vi "RealSense_HelloWorld_Left_Right_IR.vi"() -> ()   [LabVIEW 2017]
doc: "This demo shows how to connect a RealSense D4xx Stereo Depth Camera, and stream the LEFT and the RIGHT raw unrectified images."
uses:
  libRealSense3.lvlib
panel:
  in  "Zoom Factor":sgl
  in  "AutoZoom":bool
  out "Output stream format":T1
  in  "laser on/off":bool
  out "Left IR":picture
  out "Right IR":picture
  out "iteration":i32
  in  "stop":bool=TRUE
  out "release frame error":string="No Error"
  out "Capture1 Error":string="No Error"
  out "Config error":string="No Error\rNo Error"
  out "init results":T2={"camera name"="Intel RealSense 415", "camera S/N"="725112060291", "F/W"="05.08.09.00", "Sensor name"="Stereo Module", "api_version"=20710, "rscontext"=659718592, "device_list"=396628960, "device count"=2, "Dev out"=662505184, "sensor_list"=395031584, "sensor count"=2, "Sensor out"=662178704}
  out "init error":string="No Error\rNo Error\rNo Error\rNo Error\rNo Error\rNo Error\rNo Error\rNo Error\rNo Error\rNo Error\rNo Error"
  out "Close Error":string="No Error\rNo Error\rNo Error\rNo Error"
  out "Start Error":string="No Error\rNo Error\rNo Error"
  out "Capture2 error":string="No Error"
  in  "Select Resolution":u16(ring)=3 items=["256 x 144 @90fps", "424 x 240 @6fps", "424 x 240 @15fps", "424 x 240 @30fps", "424 x 240 @60fps", "424 x 240 @90fps", "480 x 270 @6fps", "480 x 270 @15fps", "480 x 270 @30fps", "480 x 270 @60fps", "480 x 270 @90fps", "640 x 360 @6fps", "640 x 360 @15fps", "640 x 360 @30fps", "640 x 360 @60fps", "640 x 360 @90fps", "640 x 480 @6fps", "640 x 480 @15fps", "640 x 480 @30fps", "640 x 480 @60fps", "640 x 480 @90fps", "848 x 100 @100fps", "848 x 480 @6fps", "848 x 480 @15fps", "848 x 480 @30fps", "848 x 480 @60fps", "848 x 480 @90fps", "1280 x 720 @6fps", "1280 x 720 @15fps", "1280 x 720 @30fps", "1280 x 800 @15fps", "1280 x 800 @30fps"]
  # "RealSense Hello World: Left-Right Rectified"
  # "This demo shows how to connect a RealSense D4xx Stereo Depth Camera, and stream the LEFT and the RIGHT images."
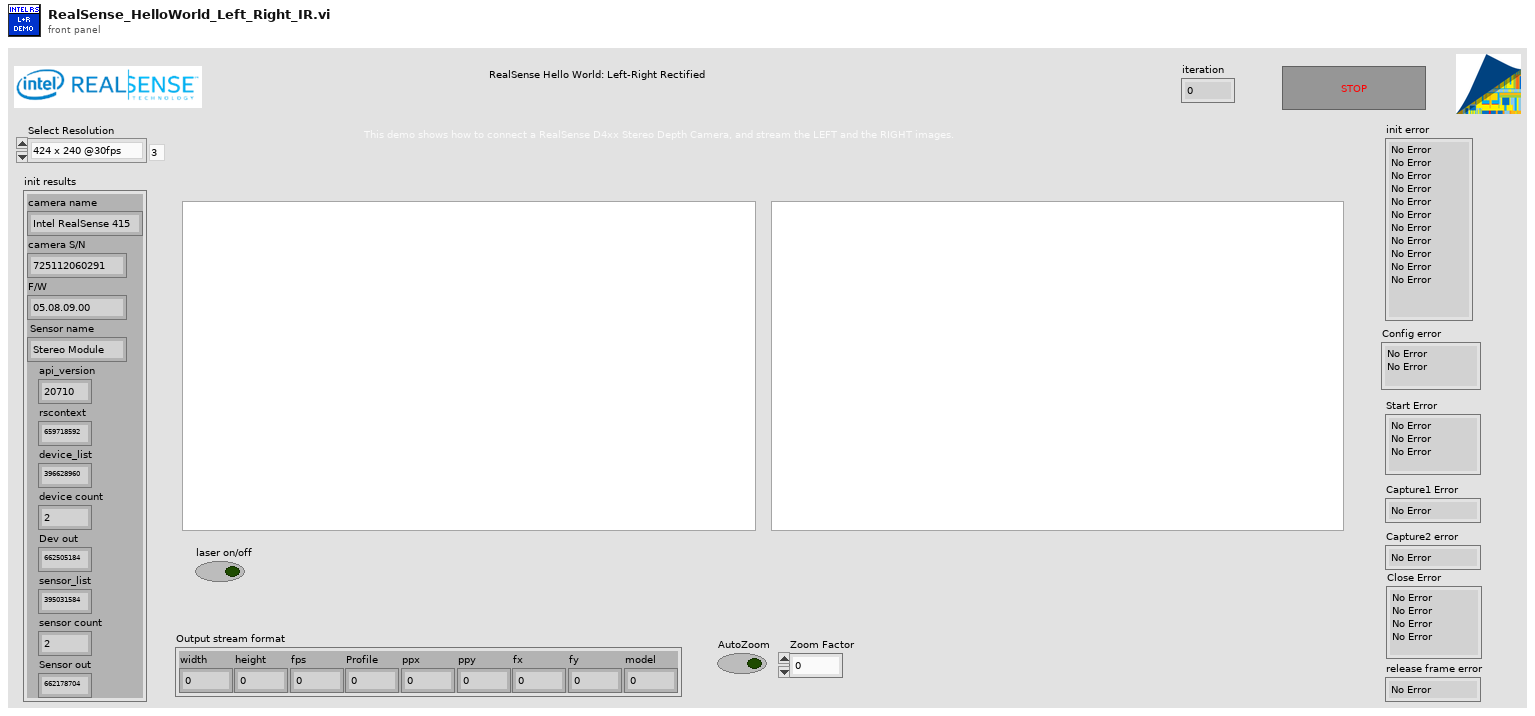
[diagram p1: front panel]
types:
  T1 = cluster{"width":i32, "height":i32, "fps":i32, "Profile":u64, "ppx":sgl, "ppy":sgl, "fx":sgl, "fy":sgl, "model":u32}
  T2 = cluster{"camera name":string, "camera S/N":string, "F/W":string, "Sensor name":string, "api_version":i32, "rscontext":u64, "device_list":u64, "device count":i32, "Dev out":u64, "sensor_list":u64, "sensor count":i32, "Sensor out":u64}
  T3 = enum16{"Depth", "Color (ext.)", "Color (left) ", "IR Left", "IR Right", "IR Left (Y16)", "IR Right (Y16)"}
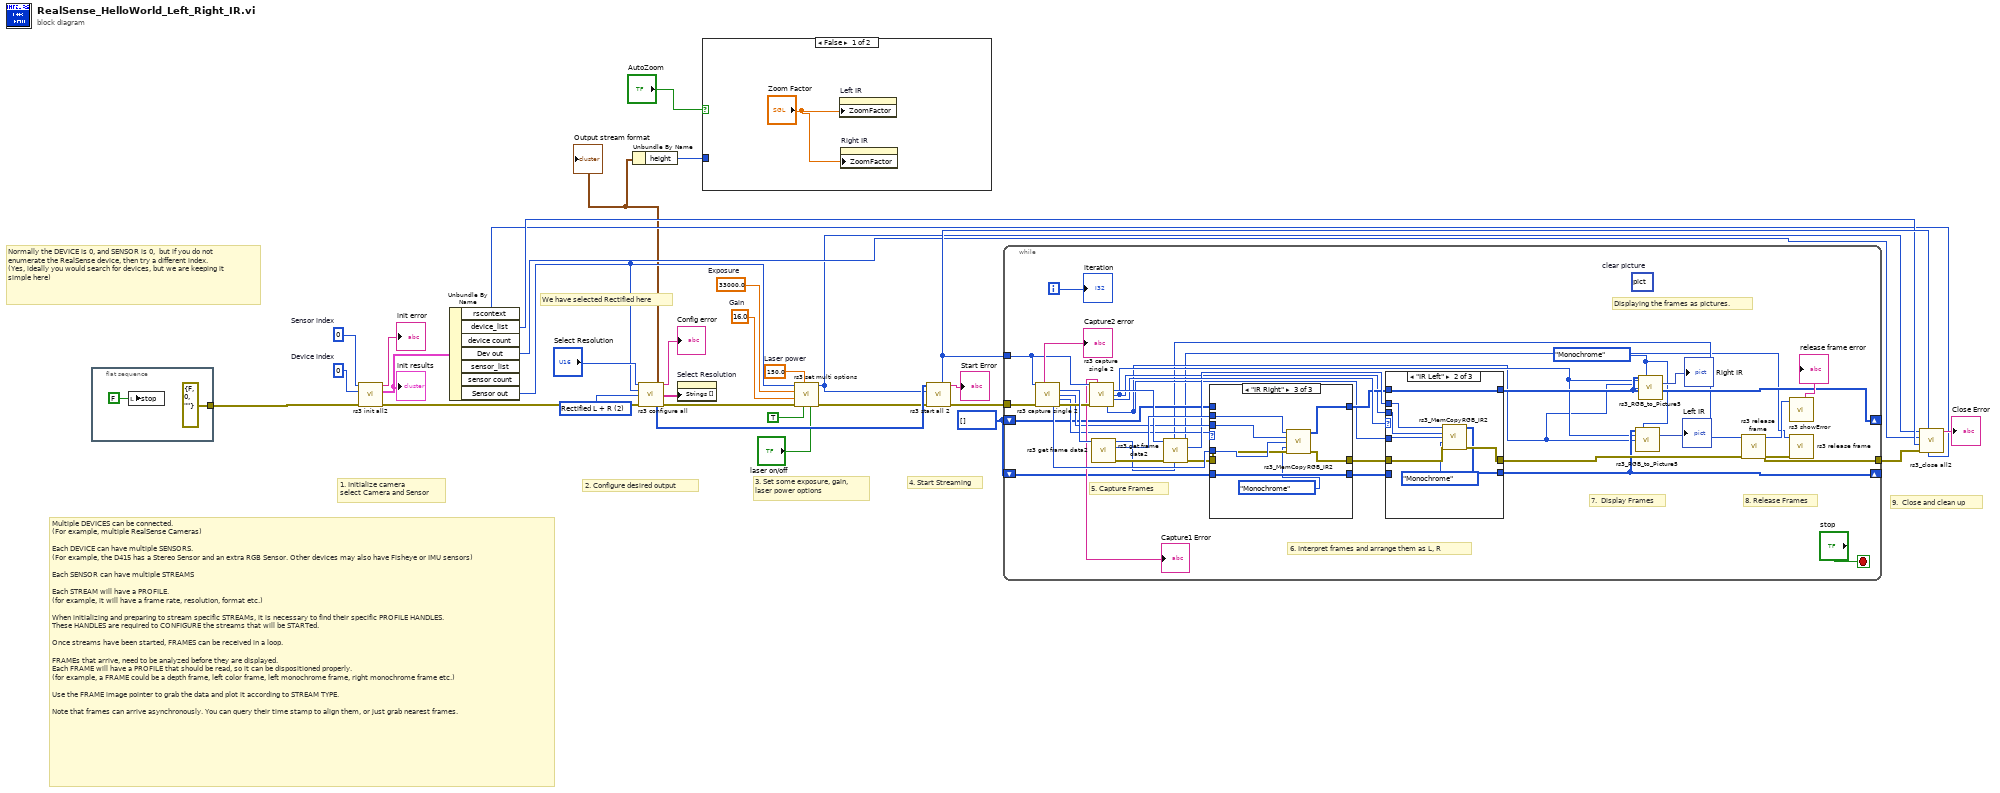
[diagram p0: block diagram]
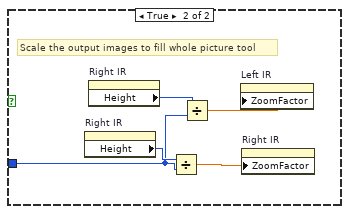
[diagram p2: hidden frame]
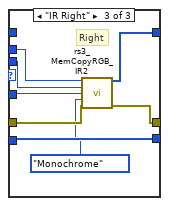
[diagram p4: hidden frame]
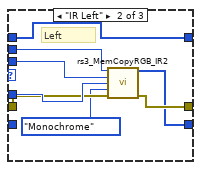
[diagram p6: hidden frame]
diagram:
  w2 = u16 2 items=["Depth + Left Color", "Unrectified L + R", "Rectified L + R", "Depth Only", "RGB ext. Only", "Depth + L Monochrome"] ("Stream selection")
  w6 = u8[] [] ("Output Array")
  w32 = 0  # Device index
  w31 = 0  # Sensor index
  w8 = sgl 16.0  # Gain
  w9 = sgl 150.0  # Laser power
  w10 = sgl 33000.0  # Exposure
  # "We have selected Rectified here"
  # "Normally the DEVICE is 0, and SENSOR is 0,  but if you do not enumerate the RealSense device, then try a different index.\n(Yes, ideally you would search for devices, but we are keeping it simple here)"
  # "Multiple DEVICES can be connected. \n(For example, multiple RealSense Cameras)\n\nEach DEVICE can have multiple SENSORS. \n(For example, the D415 has a Stereo Sensor and an extra RGB Sensor. Other devices may also have Fisheye or IMU sensors) \n\nEach SENSOR can have multiple STREAMS\n\nEach STREAM will have a PROFILE. \n(for example, it will have a frame rate, resolution, format etc.)\n\nWhen initializing and preparing to stream specific STREAMs, it is necessary to find their specific PROFILE HANDLES.\nThese HANDLES are required to CONFIGURE the streams that will be STARTed. \n\nOnce streams have been started, FRAMES can be received in a loop. \n \nFRAMEs that arrive, need to be analyzed before they are displayed. \nEach FRAME will have a PROFILE that should be read, so it can be dispositioned properly.\n(for example, a FRAME could be a depth frame, left color frame, left monochrome frame, right monochrome frame etc.)\n\nUse the FRAME image pointer to grab the data and plot it according to STREAM TYPE.\n\nNote that frames can arrive asynchronously. You can query their time stamp to align them, or just grab nearest frames."
  # "9.  Close and clean up"
  # "4. Start Streaming"
  # "3. Set some exposure, gain, \nlaser power options"
  # "2. Configure desired output"
  # "1. Initialize camera\nselect Camera and Sensor"
  n1 = flat-sequence {
    tunnel: [errorcluster {"status"=FALSE, "code"=0, "source"=""} ("error in")] -> w15
    frame #0 {
      n2 = local write "stop"(FALSE ("stop")) -> ()
    }
  }
  n3 = call "rs3 init all2.vi"("error in"=w15, "Select Device"=w32, "Select Sensor"=w31) -> ("error out"=w30:errorcluster, "init results"=w23:T2, "init error"=→"init error":string)  [unwired: 2 in, 4 out]
  "init results" <- w23
  n4 = Unbundle By Name(w23) -> ("rscontext"=w21:u64, "device_list"=w22:u64, "Dev out"=w18:u64, "Sensor out"=w12:u64)  [unwired: 3 out]
  n5 = call "rs3 configure all.vi"("Select Resolution"="Select Resolution", "Sensor in"=w12, "Stream selection"=w2, "error in (no error)"=w30) -> ("Output stream L"=w4:T1, "config error"=→"Config error":string, "Output stream"=w16:string[], "Stream Profile Handles"=w29:u64[], "error out"=w14:errorcluster)  [unwired: 2 in, 5 out]
  "Output stream format" <- w4
  n6 = Unbundle By Name(w4) -> ("height"=w3:i32)
  n7 = property on="Select Resolution" class="Ring (strict)"("Strings []"=w16) -> ()  [unwired: 2 in, 2 out]
  n8 = case shown="False" "AutoZoom" {
    tunnel: w3 -> [_ w38]
    frame False {
      n9 = property on="Left IR" class="Pict"("ZoomFactor"="Zoom Factor") -> ()  [unwired: 2 in, 2 out]
      n10 = property on="Right IR" class="Pict"("ZoomFactor"="Zoom Factor") -> ()  [unwired: 2 in, 2 out]
    }
    frame True {
      # "Scale the output images to fill whole picture tool"
      n11 = property on="Right IR" class="Pict"() -> ("Height"=w40:u32)  [unwired: 2 in, 2 out]
      n12 = property on="Right IR" class="Pict"() -> ("Height"=w37:u32)  [unwired: 2 in, 2 out]
      n13 = Divide(x=w40, y=w38) -> (x/y=w39:dbl)
      n14 = Divide(x=w37, y=w38) -> (x/y=w36:dbl)
      n15 = property on="Left IR" class="Pict"("ZoomFactor"=w36) -> ()  [unwired: 2 in, 2 out]
      n16 = property on="Right IR" class="Pict"("ZoomFactor"=w39) -> ()  [unwired: 2 in, 2 out]
    }
  }
  n17 = call "rs3 set multi options.vi"("laser on/off"="laser on/off", "autoexposure"=TRUE, "Laser power, mW (0-360)"=w9, "error in (no error)"=w14, "Gain(16-248)"=w8, "Exposure, us"=w10, "Sensor in"=w12) -> ("error out"=w13:errorcluster, "Sensor out"=w11:u64)  [unwired: 2 in, 1 out]
  n18 = call "rs3 start all 2.vi"("error in (no error)"=w13, "Sensor in"=w11, "Stream profile array"=w29) -> ("error out"=w17:errorcluster, "Config Error"=→"Start Error":string, "queue out"=w28:u64)  [unwired: 5 in, 1 out]
  n19 = while {
    tunnel: w28 -> [w65]
    tunnel: w17 -> [w76]
    tunnel: [w70] -> w27
    shift-right: [w48] -> _
    shift-left: w6 -> [w53]
    shift-right: [w49] -> _
    shift-left: w6 -> [w51]
    i -> [w75]
    stop <- "stop" stop-if-true
    w41 = enum16{"Monochrome", "RGB internal (RGB)"}."Monochrome" ("Color format")
    (unwired) picture bytes[33]  # clear picture
    # "Displaying the frames as pictures."
    # "8. Release Frames"
    # "7.  Display Frames"
    # "6. Interpret frames and arrange them as L, R"
    # "5. Capture Frames"
    n20 = call "rs3 capture single 2.vi"("queue in"=w65, "error in (no error)"=w76) -> ("Capture Error"=→"Capture2 error":string, "frame out"=w74:u64, "width"=w62:i32, "Stream type"=w54:T3, "height"=w72:i32, "error out"=w66:errorcluster)  [unwired: 2 in, 6 out]
    n21 = call "rs3 capture single 2.vi"("queue in"=w65, "error in (no error)"=w66) -> ("Capture Error"=→"Capture1 Error":string, "frame out"=w63:u64, "width"=w47:i32, "Stream type"=w56:T3, "height"=w46:i32)  [unwired: 2 in, 7 out]
    n22 = call "rs3 get frame data2.vi"("frame in"=w74) -> ("error out"=w69:errorcluster, "image pointer out"=w73:u64, "Frame out"=w45:u64)  [unwired: 7 in, 1 out]
    n23 = call "rs3 get frame data2.vi"("error in (no error)"=w69, "frame in"=w63) -> ("error out"=w68:errorcluster, "image pointer out"=w55:u64, "Frame out"=w44:u64)  [unwired: 6 in, 1 out]
    n24 = case shown="\"IR Right\"" w54 {
      tunnel: [w98 w102 w110] -> w58
      tunnel: w73 -> [_ w106 w114]
      tunnel: w62 -> [_ w105 w113]
      tunnel: w72 -> [_ w104 w112]
      tunnel: w68 -> [w98 w103 w111]
      tunnel: [w97 w101 w109] -> w52
      tunnel: w53 -> [w97 _ w109]
      tunnel: w51 -> [w96 w100 _]
      tunnel: [w96 w100 w108] -> w50
      frame "Color (ext.)", Default {
      }
      frame "IR Left" {
        # "Left"
        n25 = call "rs3_MemCopyRGB_IR2.vi"("Zimage pointer"=w106, "RGB  X, width"=w105, "RGB Y, height"=w104, "Color format"=enum16{"Monochrome", "RGB internal (RGB)"}."Monochrome", "error in (no error)"=w103) -> ("Output Array"=w101:u8[], "error out"=w102:errorcluster)  [unwired: 8 in, 1 out]
      }
      frame "IR Right" {
        n26 = call "rs3_MemCopyRGB_IR2.vi"("Zimage pointer"=w114, "RGB  X, width"=w113, "RGB Y, height"=w112, "Color format"=enum16{"Monochrome", "RGB internal (RGB)"}."Monochrome", "error in (no error)"=w111) -> ("Output Array"=w108:u8[], "error out"=w110:errorcluster)  [unwired: 8 in, 1 out]
      }
    }
    n27 = case shown="\"IR Left\"" w56 {
      tunnel: [w79 w85 w92] -> w57
      tunnel: w55 -> [_ w87 w95]
      tunnel: w47 -> [_ w83 w90]
      tunnel: w46 -> [_ w84 w91]
      tunnel: w58 -> [w79 w86 w93]
      tunnel: w52 -> [w77 _ w89]
      tunnel: w50 -> [w78 w82 _]
      tunnel: [w78 w82 w94] -> w49
      tunnel: [w77 w81 w89] -> w48
      frame "Color (ext.)", Default {
      }
      frame "IR Left" {
        n28 = call "rs3_MemCopyRGB_IR2.vi"("Zimage pointer"=w87, "RGB  X, width"=w83, "RGB Y, height"=w84, "Color format"=enum16{"Monochrome", "RGB internal (RGB)"}."Monochrome", "error in (no error)"=w86) -> ("Output Array"=w81:u8[], "error out"=w85:errorcluster)  [unwired: 8 in, 1 out]
      }
      frame "IR Right" {
        # "Right"
        n29 = call "rs3_MemCopyRGB_IR2.vi"("Zimage pointer"=w95, "RGB  X, width"=w90, "RGB Y, height"=w91, "Color format"=enum16{"Monochrome", "RGB internal (RGB)"}."Monochrome", "error in (no error)"=w93) -> ("Output Array"=w94:u8[], "error out"=w92:errorcluster)  [unwired: 8 in, 1 out]
      }
    }
    n30 = call "rs3_RGB_to_Picture5.vi"("RGB array"=w48, "Color format"=w41, "RGB  X, width"=w47, "RGB Y, height"=w46) -> ("new picture"=→"Left IR":picture)  [unwired: 10 in, 1 out]
    n31 = call "rs3_RGB_to_Picture5.vi"("RGB array"=w49, "Color format"=w41, "RGB  X, width"=w47, "RGB Y, height"=w46) -> ("new picture"=→"Right IR":picture)  [unwired: 10 in, 1 out]
    n32 = call "rs3 release frame.vi"("error in (no error)"=w57, "Frame"=w45) -> ("error out"=w71:errorcluster, "error"=w61:u64)  [unwired: 8 in]
    n33 = call "rs3 showError.vi"("error"=w61) -> ("Error summary"=→"release frame error":string)  [unwired: 6 in, 4 out]
    n34 = call "rs3 release frame.vi"("error in (no error)"=w71, "Frame"=w44) -> ("error out"=w70:errorcluster)  [unwired: 8 in, 1 out]
    "iteration" <- w75
  }
  n35 = call "rs3_close all2.vi"("rscontext"=w21, "queue in"=w28, "error in (no error)"=w27, "device_list"=w22, "Dev in"=w18, "Sensor in"=w11) -> ("Close Error"=→"Close Error":string)  [unwired: 4 in, 1 out]
